vi "Set.vi"(8 "error in (no error)":errorcluster, 9 "status in":T1 items=["Closed", "Open"], 10 "valve in":T2 items=["Valve 1"=1, "Valve 2"=2, "Valve 3"=3, "Valve 4"=4, "Valve 5"=5, "Valve 6"=6, "Valve 7"=7], 11 "Valve Controller in":refnum<class "Valve Controller.lvclass">) -> (0 "error out":errorcluster, 1 "status out":T1 items=["Closed", "Open"], 2 "Valve out":T2=7 items=["Valve 1"=1, "Valve 2"=2, "Valve 3"=3, "Valve 4"=4, "Valve 5"=5, "Valve 6"=6, "Valve 7"=7], 3 "Valve Controller out":refnum<class "Valve Controller.lvclass">)   [LabVIEW 2011, in "Valve Controller.lvclass"]
uses:
  Valve Controller.lvclass
  Valves.ctl
  Status.ctl
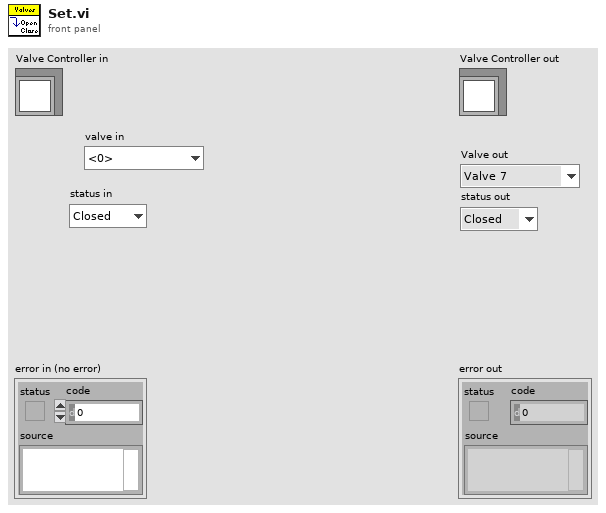
[diagram p1: front panel]
types:
  T1 = typedef "Valve Controller.lvclass/Status.ctl" = u16
  T2 = typedef "Valve Controller.lvclass/Valves.ctl" = u16
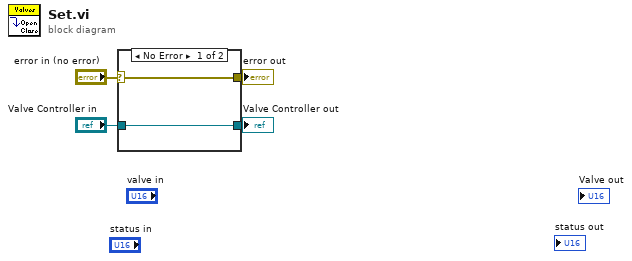
[diagram p0: block diagram]
diagram:
  n1 = case shown="No Error" "error in (no error)" {
    selector: "error in (no error)" -> [w5 w8]
    tunnel: [w5 w8] -> w3
    tunnel: [w6 w7] -> w1
    tunnel: "Valve Controller in" -> [w6 w7]
    frame No Error {
    }
    frame Error {
    }
  }
  "error out" <- w3
  "Valve Controller out" <- w1
